vi "1A Helper - UTC to TimeStamp.vi"(4 "UTC Time Zone in":i32=-5, 5 "UTC (hhmmss)":string) -> (1 "Local Time":timestamp, 2 "UTC Time":timestamp)   [LabVIEW 2011]
doc: "This VI parses UTC (hhmmss) string time data from a GPS and combines it with the current date data from the platform (computer or RIO) to get UTC and Local Timestamps."
uses:
  <vilib>/Utility/miscctls.llb/LVDateTimeRec.ctl
  <vilib>/regexp/Match Regular Expression.xnode
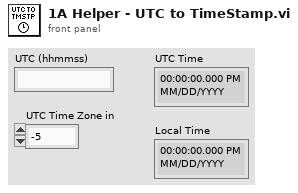
[diagram p1: front panel]
types:
  T1 = typedef "LVDateTimeRec.ctl" = cluster{"fractional second":dbl, "second":i32, "minute":i32, "hour":i32, "day of month":i32, "month":i32, "year":i32, "day of week":i32, "day of year":i32, "DST":i32}
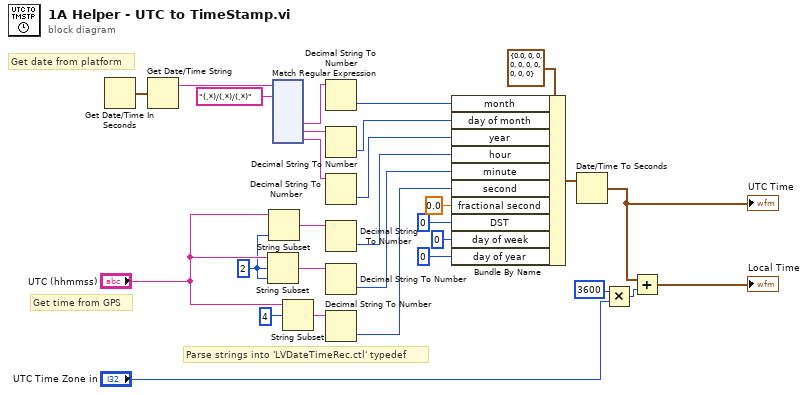
[diagram p0: block diagram]
diagram:
  w5 = 2 ("length (rest)")
  # "Parse strings into 'LVDateTimeRec.ctl' typedef"
  # "Get time from GPS"
  # "Get date from platform"
  n1 = Get Date/Time In Seconds() -> (seconds since 1Jan1904=w1:timestamp)
  n2 = Get Date/Time String(seconds (now)=w1) -> (date string=w10:string)  [unwired: 2 in, 1 out]
  n3 = String Subset(string="UTC (hhmmss)", offset (0)=w5, length (rest)=w5) -> (substring=w4:string)
  n4 = String Subset(string="UTC (hhmmss)", length (rest)=w5) -> (substring=w6:string)  [unwired: 1 in]
  n5 = xnode "Match Regular Expression"("input string"=w10, "regular expression"="(.*)/(.*)/(.*)") -> ("submatch 1"=w12:string, "submatch 2"=w13:string, "submatch 3"=w14:string)  [unwired: 4 in, 5 out]
  n6 = String Subset(string="UTC (hhmmss)", offset (0)=4) -> (substring=w2:string)  [unwired: 1 in]
  n7 = Decimal String To Number(string=w12) -> (number=w15:i32)  [unwired: 2 in, 1 out]
  n8 = Decimal String To Number(string=w13) -> (number=w16:i32)  [unwired: 2 in, 1 out]
  n9 = Decimal String To Number(string=w14) -> (number=w17:i32)  [unwired: 2 in, 1 out]
  n10 = Decimal String To Number(string=w6) -> (number=w7:i32)  [unwired: 2 in, 1 out]
  n11 = Decimal String To Number(string=w4) -> (number=w8:i32)  [unwired: 2 in, 1 out]
  n12 = Decimal String To Number(string=w2) -> (number=w9:i32)  [unwired: 2 in, 1 out]
  n13 = Bundle By Name(cluster=T1 {"fractional second"=0.0, "second"=0, "minute"=0, "hour"=0, "day of month"=0, "month"=0, "year"=0, "day of week"=0, "day of year"=0, "DST"=0} ("date time rec"), "month"=w15, "day of month"=w16, "year"=w17, "hour"=w7, "minute"=w8, "second"=w9, "fractional second"=0.0, "DST"=0, "day of week"=0, "day of year"=0) -> (w19:T1)
  n14 = Date/Time To Seconds(2:w19) -> (0:w29:timestamp)  [unwired: 1 in]
  "UTC Time" <- w29
  n15 = Multiply(x=3600 ("number"), y="UTC Time Zone in") -> (x*y=w27:i32)
  n16 = Add(x=w29, y=w27) -> (x+y=→"Local Time":timestamp)
